vi "S2C_About.vi"(8 "Error In":errorcluster) -> (0 "Error Out":errorcluster)   [LabVIEW 2015]
doc: "Prompt used to display the current revision of the application software."
panel:
  in  "String":string="Script 2 Code Engine (S2Ce)\n\nRevision 1.00.00"
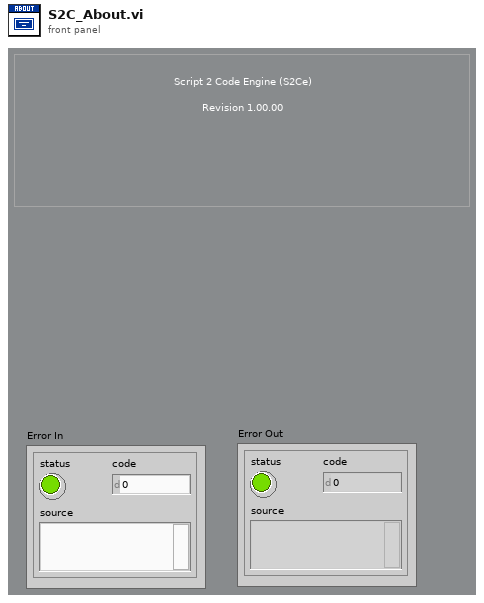
[diagram p1: front panel]
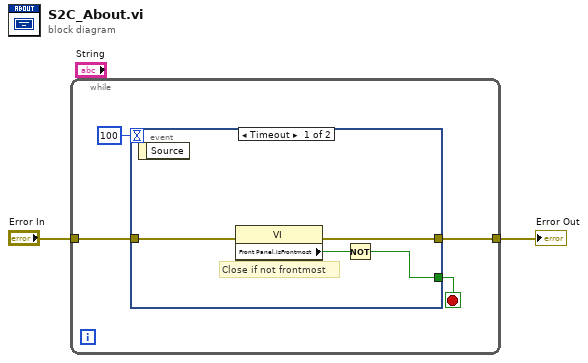
[diagram p0: block diagram]
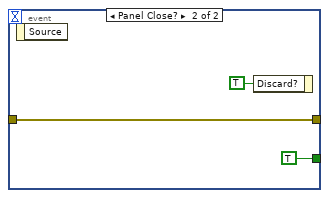
[diagram p2: hidden frame]
diagram:
  n1 = while {
    tunnel: "Error In" -> [w6]
    tunnel: [w5] -> w2
    stop <- w4 stop-if-true
    n2 = event shown="[0] Timeout" {
      selector: _ -> [_ _]
      dyn-events: _ -> [_ _]
      timeout: 100 -> [_ _]
      tunnel: w6 -> [w10 w13]
      tunnel: [w7 w13] -> w5
      tunnel: [w8 TRUE] -> w4
      event Timeout {
        # "Close if not frontmost"
        n3 = event-data() -> ()  [unwired: 1 in, 1 out]
        n4 = property class="VI"(error in=w10) -> (error out=w7:errorcluster, "Front Panel.IsFrontmost"=w9:bool)  [unwired: 1 in, 1 out]
        n5 = Not(x=w9) -> (.not. x?=w8:bool)
      }
      event Panel Close? {
        n6 = event-data() -> ()  [unwired: 1 in, 1 out]
        n7 = event-data("Discard?"=TRUE) -> ()  [unwired: 1 in, 1 out]
      }
    }
  }
  "Error Out" <- w2
